vi "Anthony-Sandoval-Lab2.vi"() -> ()   [LabVIEW 2010]
uses:
  <vilib>/Utility/file.llb/Write To Spreadsheet File (DBL).vi
  <vilib>/Analysis/NI_AALBase.lvlib
panel:
  in  "Save (LED ON)":bool
  out "Histogram":T1(graph)
  in  "Histogram Intervals":dbl
  in  "Number of Random numbers":i32
  out "Waveform Graph":dbl[](graph)
  in  "Expected Number":dbl
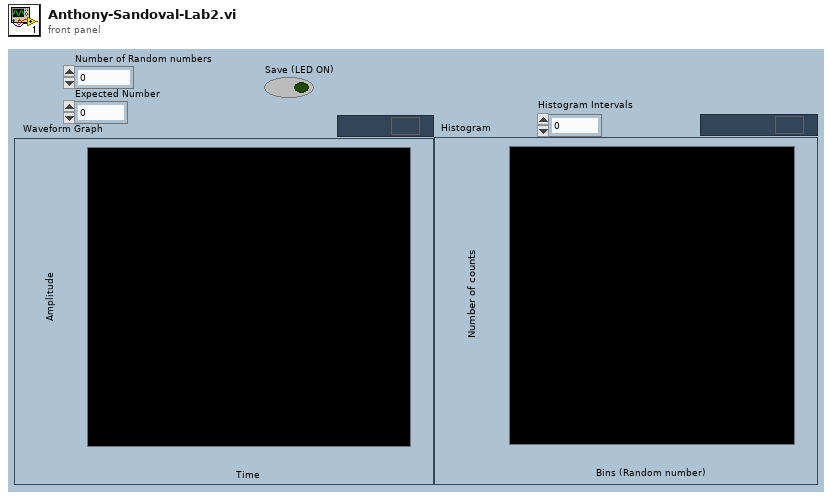
[diagram p1: front panel]
types:
  T1 = cluster{"X Values":dbl[], "Histogram: h(x)":i32[]}
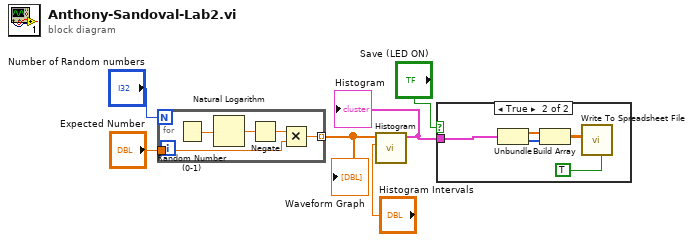
[diagram p0: block diagram]
diagram:
  n1 = for {
    N: "Number of Random numbers" -> [_]
    tunnel: "Expected Number" -> [w8]
    tunnel: [w7] -> w1 mode=indexing
    n2 = Random Number (0-1)() -> (number: 0 to 1=w10:dbl)
    n3 = Natural Logarithm(1:w10) -> (0:w11:dbl)
    n4 = Negate(x=w11) -> (-x=w9:dbl)
    n5 = Multiply(x=w9, y=w8) -> (x*y=w7:dbl)
  }
  "Waveform Graph" <- w1
  n6 = call <vilib>:"Histogram.vi"("intervals"="Histogram Intervals", "X"=w1) -> ("Histogram Graph"=w3:T1)  [unwired: 6 in, 3 out]
  "Histogram" <- w3
  n7 = case shown="True" "Save (LED ON)" {
    tunnel: w3 -> [_ w16]
    frame False {
    }
    frame True {
      n8 = Unbundle(w16) -> ("X Values"=w14:dbl[], "Histogram: h(x)"=w15:i32[])
      n9 = Build Array(w14, w15) -> (w13:dbl[][])
      n10 = call-poly <vilib>:"Write To Spreadsheet File.vi"("transpose? (no:F)"=TRUE, "2D data"=w13) -> ()  [unwired: 6 in, 1 out]
    }
  }
